vi "McPherson Set Speed.vi"(0 "PS Communication Port":T1=1 items=["Modem", "Printer", "COM3", "COM4", "COM5", "COM6", "COM7", "COM8", "COM9", "Nothing", "LPT1", "LPT2", "LPT3", "LPT4"], 2 "ScanSpeed In":i16, 3 "error In":errorcluster, 4 "Scan(F)orStop(T)":bool) -> (5 "ScanSpeed Out":i32, 6 "error out":errorcluster)   [LabVIEW 2019]
uses:
  Serial Instruments/Serial Support VISA.llb/Communication Port.ctl
  Globals and TypeDefs/Global Varibal Control.vi
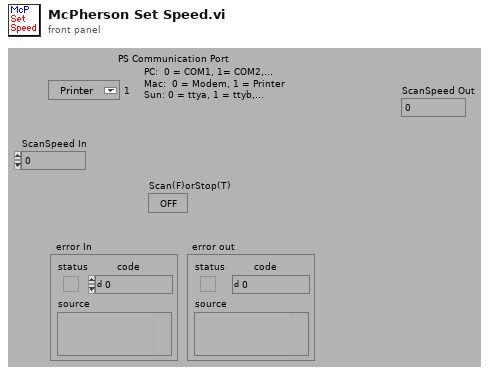
[diagram p1: front panel]
types:
  T1 = typedef "Communication Port.ctl" = u16
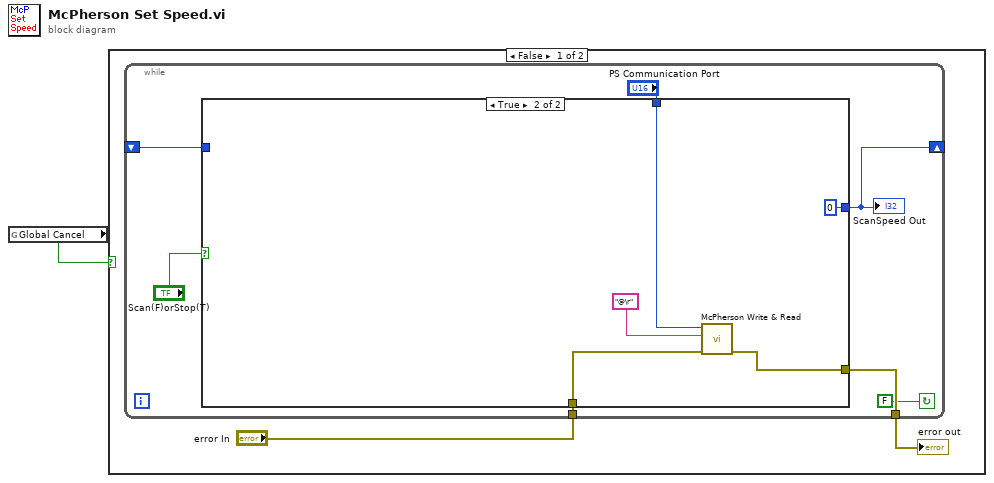
[diagram p0: block diagram]
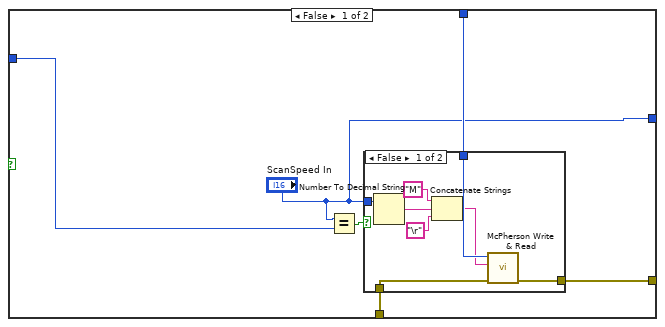
[diagram p2: hidden frame]
diagram:
  n1 = global read "Global Varibal Control.vi" "Global Cancel"() -> (w1:bool)
  n2 = case shown="False" w1 {
    frame False {
      n3 = while {
        shift-left: _ -> [w5]
        shift-right: [w6] -> _
        tunnel: "error In" -> [w9]
        tunnel: [w10] -> w3
        stop <- FALSE continue-if-true
        n4 = case shown="True" "Scan(F)orStop(T)" {
          tunnel: [w16 w29] -> w10
          tunnel: w9 -> [w15 w30]
          tunnel: "PS Communication Port" -> [w14 w28]
          tunnel: ["ScanSpeed In" i16 0] -> w6
          tunnel: w5 -> [w11 _]
          frame False {
            n5 = Equal?(x="ScanSpeed In", y=w11) -> (x = y?=w12:bool)
            n6 = case shown="False" w12 {
              tunnel: [w24 w25] -> w16
              tunnel: w15 -> [w23 w25]
              tunnel: w14 -> [w22 _]
              tunnel: "ScanSpeed In" -> [w17 _]
              frame False {
                n7 = Number To Decimal String(number=w17) -> (decimal integer string=w20:string)  [unwired: 1 in]
                n8 = Concatenate Strings("M" ("Substring"), w20, "\r" ("Substring")) -> (w18:string)
                n9 = call "McPherson Write & Read.vi"("error in (no error)"=w23, "Write String"=w18, "PortNumber"=w22) -> ("error out"=w24:errorcluster)  [unwired: 2 in, 3 out]
              }
              frame True {
              }
            }
          }
          frame True {
            n10 = call "McPherson Write & Read.vi"("error in (no error)"=w30, "Write String"="@\r" ("Substring"), "PortNumber"=w28) -> ("error out"=w29:errorcluster)  [unwired: 2 in, 3 out]
          }
        }
        "ScanSpeed Out" <- w6
      }
      "error out" <- w3
    }
    frame True {
    }
  }
